vi "Setup camera parameters.vi"(8 "error in (no error)":errorcluster, 11 "Retiga in":refnum<class "Retiga.lvclass">) -> (0 "error out":errorcluster, 3 "Retiga out":refnum<class "Retiga.lvclass">)   [LabVIEW 2012, in "Retiga.lvclass"]
uses:
  Retiga.lvclass
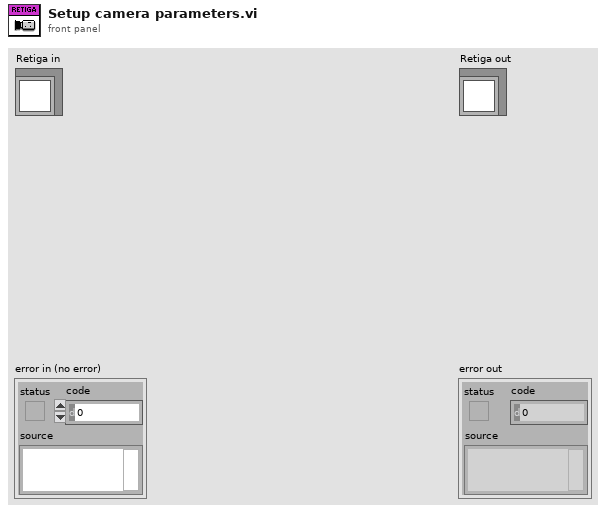
[diagram p1: front panel]
types:
  T1 = enum32{"gain", "offset", "exposure", "binning", "horizontal binning", "vertical binning", "readout speed", "trigger type", "lcd filter", "cooler", "exposure red", "exposure blue", "image format", "roi x", "roi y", "roi width", "roi height", "reserved1", "shutter state", "reserved2", "sync-b out", "reserved3", "intensifier gain", "trigger delay", "camera mode", "normalized gain", "normalized intenifier gain DB", "doPostProcessing", "postProcessGainRed", "postProcessGainGreen", "postProcessGainBlue", "postProcessBayerAlgorithm", "postProcessImageFormat", "fan", "blackout mode", "high sensitivity", "Readout Port", "EM Gain", "open delay", "close delay", "clearing mode"}
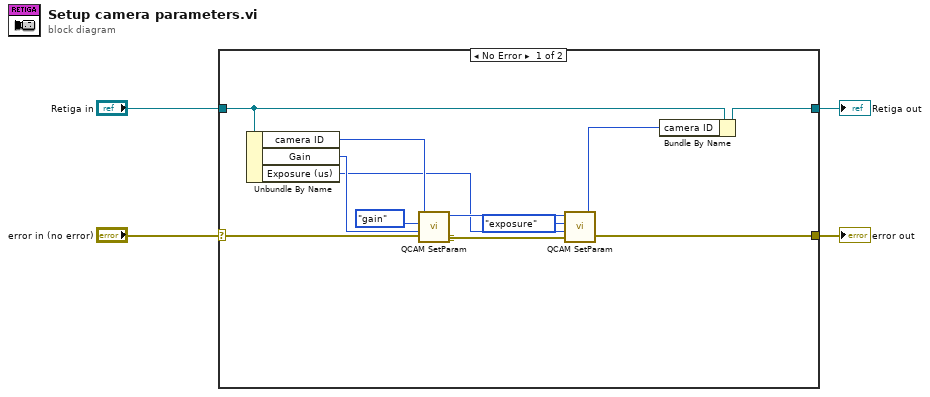
[diagram p0: block diagram]
diagram:
  n1 = case shown="No Error" "error in (no error)" {
    selector: "error in (no error)" -> [w9 w18]
    tunnel: [w8 w18] -> w3
    tunnel: [w6 w17] -> w1
    tunnel: "Retiga in" -> [w7 w17]
    frame No Error {
      n2 = Unbundle By Name(w7) -> ("camera ID"=w15:u32, "Gain"=w14:i32, "Exposure (us)"=w11:i32)
      n3 = call <userlib>:"QCAM SetParam.vi"("error in (no error)"=w9, "value"=w14, "parameter key"=T1."gain", "cameraId"=w15) -> ("error out"=w12:errorcluster, "cameraId out"=w13:u32)
      n4 = call <userlib>:"QCAM SetParam.vi"("error in (no error)"=w12, "value"=w11, "parameter key"=T1."exposure", "cameraId"=w13) -> ("error out"=w8:errorcluster, "cameraId out"=w5:u32)
      n5 = Bundle By Name(cluster=w7, "camera ID"=w5) -> (w6:refnum<class "Retiga.lvclass">)
    }
    frame Error {
    }
  }
  "error out" <- w3
  "Retiga out" <- w1
